vi "Position Relative to Tunnel.vi"(7 "Tunnel Position":enum16{"Left", "Top", "Right", "Bottom"}(ring), 11 "Tunnel in":refnum<vi>) -> (2 "Inner Position":T1, 3 "Outer Position":T1)   [LabVIEW 2023]
doc: "Gives offset positions for placement of new objects on FP depending on where on the structure the tunnel lies.\n\nThe input reference type is Gobj, to allow different tunnel types to be used.\n\nThese re baseline positions, but the placed bundlers will resize when the lables are atacjed to the terminals, so to fine tune the alignment, we don't do that here. We ahve to realign after objects are in their finished state."
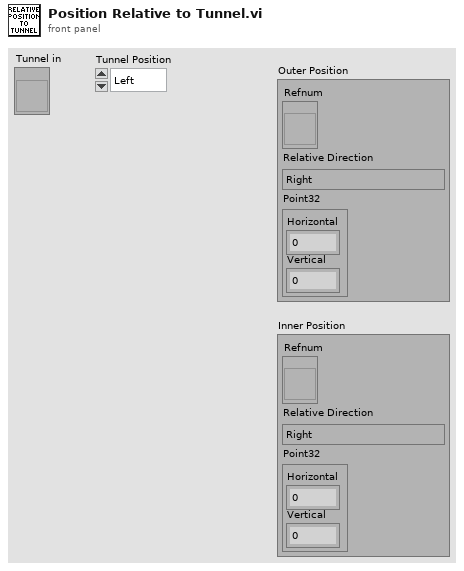
[diagram p1: front panel]
types:
  T1 = cluster{"Refnum":refnum<vi>, "Relative Direction":enum32{"Right", "Left", "Top", "Bottom", "Top Right", "Top Left", "Bottom Right", "Bottom Left"}, "Point32":cluster{"Horizontal":i32, "Vertical":i32}}
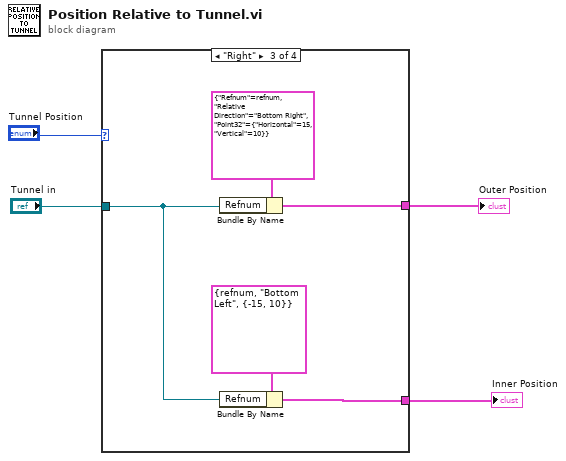
[diagram p0: block diagram]
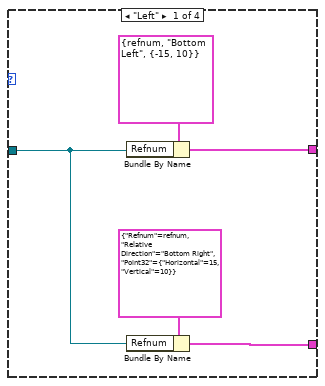
[diagram p2: hidden frame]
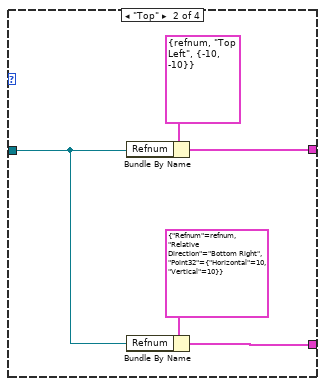
[diagram p3: hidden frame]
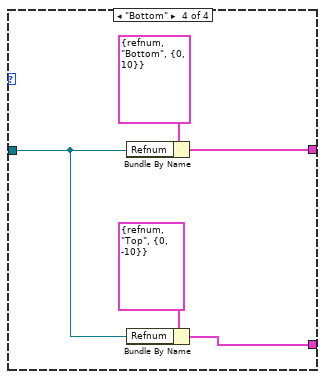
[diagram p4: hidden frame]
diagram:
  n1 = case shown="\"Right\"" "Tunnel Position" {
    tunnel: [w9 w14 w19 w24] -> w4
    tunnel: "Tunnel in" -> [w8 w13 w18 w23]
    tunnel: [w6 w11 w16 w21] -> w2
    frame "Left" {
      n2 = Bundle By Name(cluster=T1 {"Refnum"=refnum, "Relative Direction"=enum."Bottom Left", "Point32"={"Horizontal"=-15, "Vertical"=10}} ("Relative Position"), "Refnum"=w8) -> (w6:T1)
      n3 = Bundle By Name(cluster=T1 {"Refnum"=refnum, "Relative Direction"=enum."Bottom Right", "Point32"={"Horizontal"=15, "Vertical"=10}} ("Relative Position"), "Refnum"=w8) -> (w9:T1)
    }
    frame "Top" {
      n4 = Bundle By Name(cluster=T1 {"Refnum"=refnum, "Relative Direction"=enum."Top Left", "Point32"={"Horizontal"=-10, "Vertical"=-10}} ("Relative Position"), "Refnum"=w13) -> (w11:T1)
      n5 = Bundle By Name(cluster=T1 {"Refnum"=refnum, "Relative Direction"=enum."Bottom Right", "Point32"={"Horizontal"=10, "Vertical"=10}} ("Relative Position"), "Refnum"=w13) -> (w14:T1)
    }
    frame "Right" {
      n6 = Bundle By Name(cluster=T1 {"Refnum"=refnum, "Relative Direction"=enum."Bottom Right", "Point32"={"Horizontal"=15, "Vertical"=10}} ("Relative Position"), "Refnum"=w18) -> (w16:T1)
      n7 = Bundle By Name(cluster=T1 {"Refnum"=refnum, "Relative Direction"=enum."Bottom Left", "Point32"={"Horizontal"=-15, "Vertical"=10}} ("Relative Position"), "Refnum"=w18) -> (w19:T1)
    }
    frame "Bottom" {
      n8 = Bundle By Name(cluster=T1 {"Refnum"=refnum, "Relative Direction"=enum."Bottom", "Point32"={"Horizontal"=0, "Vertical"=10}} ("Relative Position"), "Refnum"=w23) -> (w21:T1)
      n9 = Bundle By Name(cluster=T1 {"Refnum"=refnum, "Relative Direction"=enum."Top", "Point32"={"Horizontal"=0, "Vertical"=-10}} ("Relative Position"), "Refnum"=w23) -> (w24:T1)
    }
  }
  "Inner Position" <- w4
  "Outer Position" <- w2
